vi "FTW-ERR-Clear.vi"(1 "error to snuff":errorcluster) -> (0 "no error":errorcluster)   [LabVIEW 2012]
panel:
  # "Inputs"
  # "Outputs"
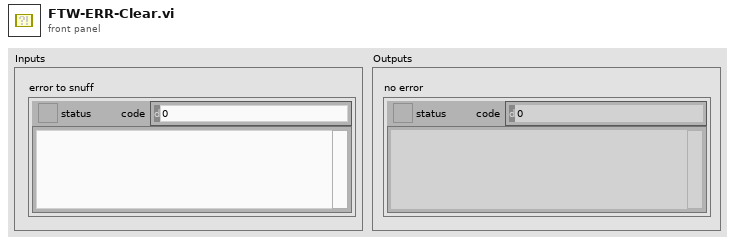
[diagram p1: front panel]
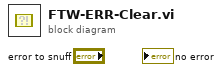
[diagram p0: block diagram]
diagram:
